vi "Write State.vi"(8 "error in (no error)":errorcluster, 10 "State":bool, 11 "Monitor in":refnum<class "Monitor.lvclass">) -> (0 "error out":errorcluster, 3 "Monitor out":refnum<class "Monitor.lvclass">)   [LabVIEW 2016, in "Monitor.lvclass"]
uses:
  Monitor.lvclass
  Monitor.lvclass/Monitor.ctl
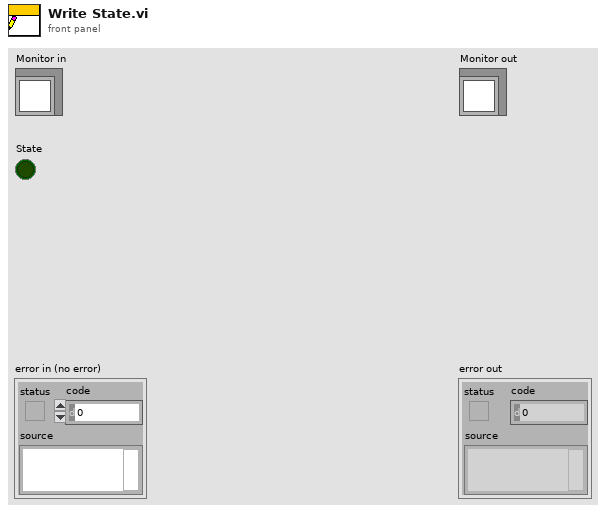
[diagram p1: front panel]
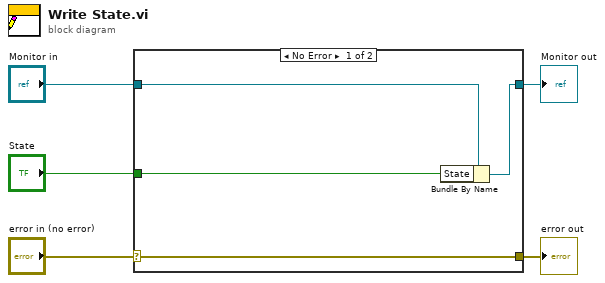
[diagram p0: block diagram]
diagram:
  n1 = case shown="No Error" "error in (no error)" {
    selector: "error in (no error)" -> [w9 w10]
    tunnel: [w9 w10] -> w4
    tunnel: [w7 w11] -> w2
    tunnel: "Monitor in" -> [w8 w11]
    tunnel: "State" -> [w6 _]
    frame No Error {
      n2 = Bundle By Name(cluster=w8, "State"=w6) -> (w7:refnum<class "Monitor.lvclass">)
    }
    frame Error {
    }
  }
  "error out" <- w4
  "Monitor out" <- w2
